vi "NF LI56xx dvr MATH calculation method.vi"(8 "error in":errorcluster caption="error in (no error)" {"code" format="%.0x"}, 9 "Read(F)":bool, 10 "set calculation \nmethod":enum16{"OFF", "EXPand", "NORMalize", "RATio"}(ring), 11 "VISA resource name":refnum<visa-resource-name>) -> (0 "error out":errorcluster {"code" format="%.0x"}, 2 "query calculation \nmethod":string, 3 "VISA resource name copy":refnum<visa-resource-name>)   [LabVIEW 2019]
doc: "Sets/queries the calculation method for measurement value to be displayed and output."
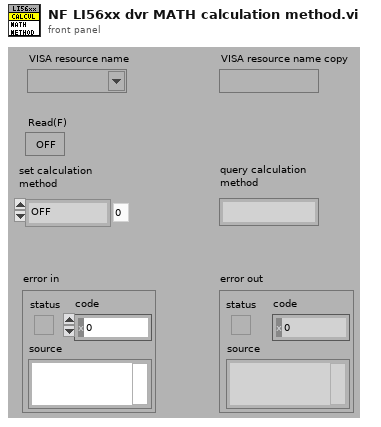
[diagram p1: front panel]
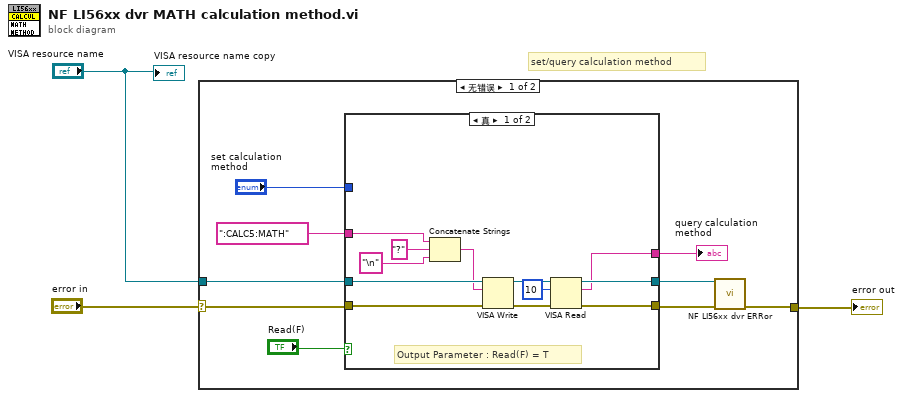
[diagram p0: block diagram]
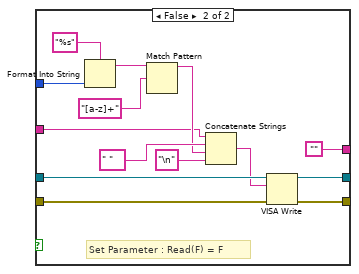
[diagram p2: hidden frame]
diagram:
  # "set/query calculation method"
  n1 = case shown="无错误" "error in" {
    selector: "error in" -> [w11 w39]
    tunnel: [w5 w39] -> w3
    tunnel: "VISA resource name" -> [w10 _]
    frame No Error {
      n2 = case shown="真" "Read(F)" {
        tunnel: w10 -> [w24 w38]
        tunnel: [w21 w35] -> w7
        tunnel: [w20 w36] -> w6
        tunnel: w11 -> [w19 w37]
        tunnel: [w15 ""] -> w9
        tunnel: "set calculation \nmethod" -> [_ w29]
        tunnel: ":CALC5:MATH" ("•¶Žš—ñ") -> [w13 w25]
        frame True {
          # "Output Parameter : Read(F) = T"
          n3 = Concatenate Strings(w13, "?" ("Œ`Ž®•¶Žš—ñ"), "\n" ("Œ`Ž®•¶Žš—ñ")) -> (w16:string)
          n4 = VISA Write(VISA resource name=w24, write buffer=w16, error in (no error)=w19) -> (VISA resource name out=w22:refnum<visa-resource-name>, error out=w23:errorcluster)  [unwired: 1 out]
          n5 = VISA Read(VISA resource name=w22, byte count=u32 10 ("バイトカウント（0）"), error in (no error)=w23) -> (VISA resource name out=w21:refnum<visa-resource-name>, read buffer=w15:string, error out=w20:errorcluster)  [unwired: 1 out]
        }
        frame False {
          # "Set Parameter : Read(F) = F"
          n6 = Format Into String(format string="%s", w29) -> (resulting string=w28:string)  [unwired: 2 in, 1 out]
          n7 = Match Pattern(string=w28, regular expression="[a-z]+") -> (before substring=w27:string)  [unwired: 1 in, 3 out]
          n8 = Concatenate Strings(w25, " ", w27, "\n" ("Œ`Ž®•¶Žš—ñ")) -> (w33:string)
          n9 = VISA Write(VISA resource name=w38, write buffer=w33, error in (no error)=w37) -> (VISA resource name out=w35:refnum<visa-resource-name>, error out=w36:errorcluster)  [unwired: 1 out]
        }
      }
      "query calculation \nmethod" <- w9
      n10 = call "NF LI56xx dvr ERRor.vi"("VISA resource name"=w7, "error in (no error)"=w6) -> ("error out"=w5:errorcluster)  [unwired: 10 in, 3 out]
    }
    frame Error {
    }
  }
  "error out" <- w3
  "VISA resource name copy" <- "VISA resource name"
